vi "test_string_tofilename.vi"(10 "Session Name/ID":string) -> (1 "fixed_name":bool, 2 "CompliantName":string)   [LabVIEW 2011]
uses:
  <vilib>/regexp/Match Regular Expression.xnode
panel:
  out "Numeric":i32
  out "whole match":string
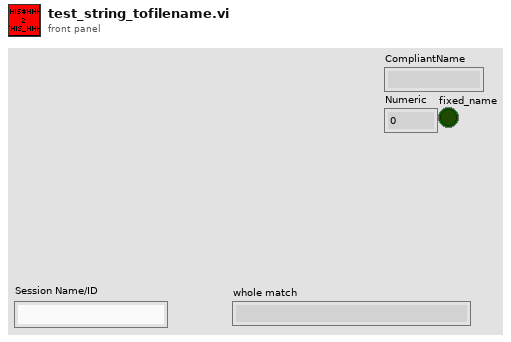
[diagram p1: front panel]
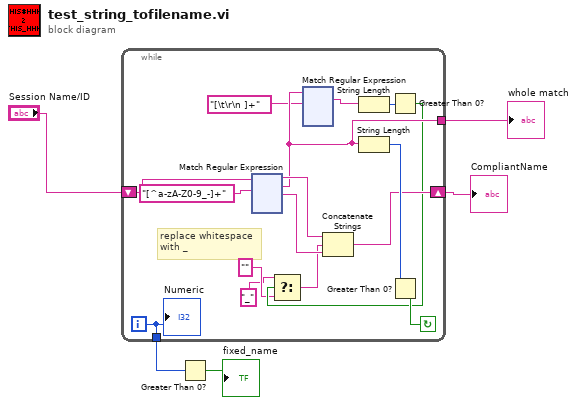
[diagram p0: block diagram]
diagram:
  n1 = while {
    tunnel: [w14] -> w5
    shift-right: [w16] -> w3
    shift-left: "Session Name/ID" -> [w20]
    tunnel: [w12] -> w2
    i -> [w12]
    stop <- w18 continue-if-true
    # "replace whitespace\nwith _"
    n2 = xnode "Match Regular Expression"("input string"=w20, "regular expression"="[^a-zA-Z0-9_-]+") -> ("before match"=w19:string, "whole match"=w14:string, "after match"=w15:string)  [unwired: 4 in, 2 out]
    n3 = xnode "Match Regular Expression"("input string"=w14, "regular expression"="[\t\r\n ]+") -> ("whole match"=w11:string)  [unwired: 4 in, 4 out]
    n4 = String Length(string=w11) -> (length=w10:i32)
    n5 = String Length(string=w14) -> (length=w17:i32)
    n6 = Greater Than 0?(x=w10) -> (x > 0?=w8:bool)
    n7 = Select(t="_", s=w8, f="") -> (s? t:f=w9:string)
    n8 = Concatenate Strings(w19, w9, w15) -> (w16:string)
    n9 = Greater Than 0?(x=w17) -> (x > 0?=w18:bool)
    "Numeric" <- w12
  }
  "whole match" <- w5
  "CompliantName" <- w3
  n10 = Greater Than 0?(x=w2) -> (x > 0?=→"fixed_name":bool)
